vi "RP read signal channel.vi"(7 "Pipeline delay":dbl=28.0, 8 "Error In":errorcluster, 9 "Channel name":string, 11 "File Path Control":path) -> (0 "Error Out":errorcluster, 1 "Phase":dbl, 2 "Frequency":dbl format="%_19p", 3 "Data out":waveform(dbl), 4 "Phase word":u32, 5 "Frequency word":u32)   [LabVIEW 2015]
panel:
  out "t0":dbl format="%#_6p"
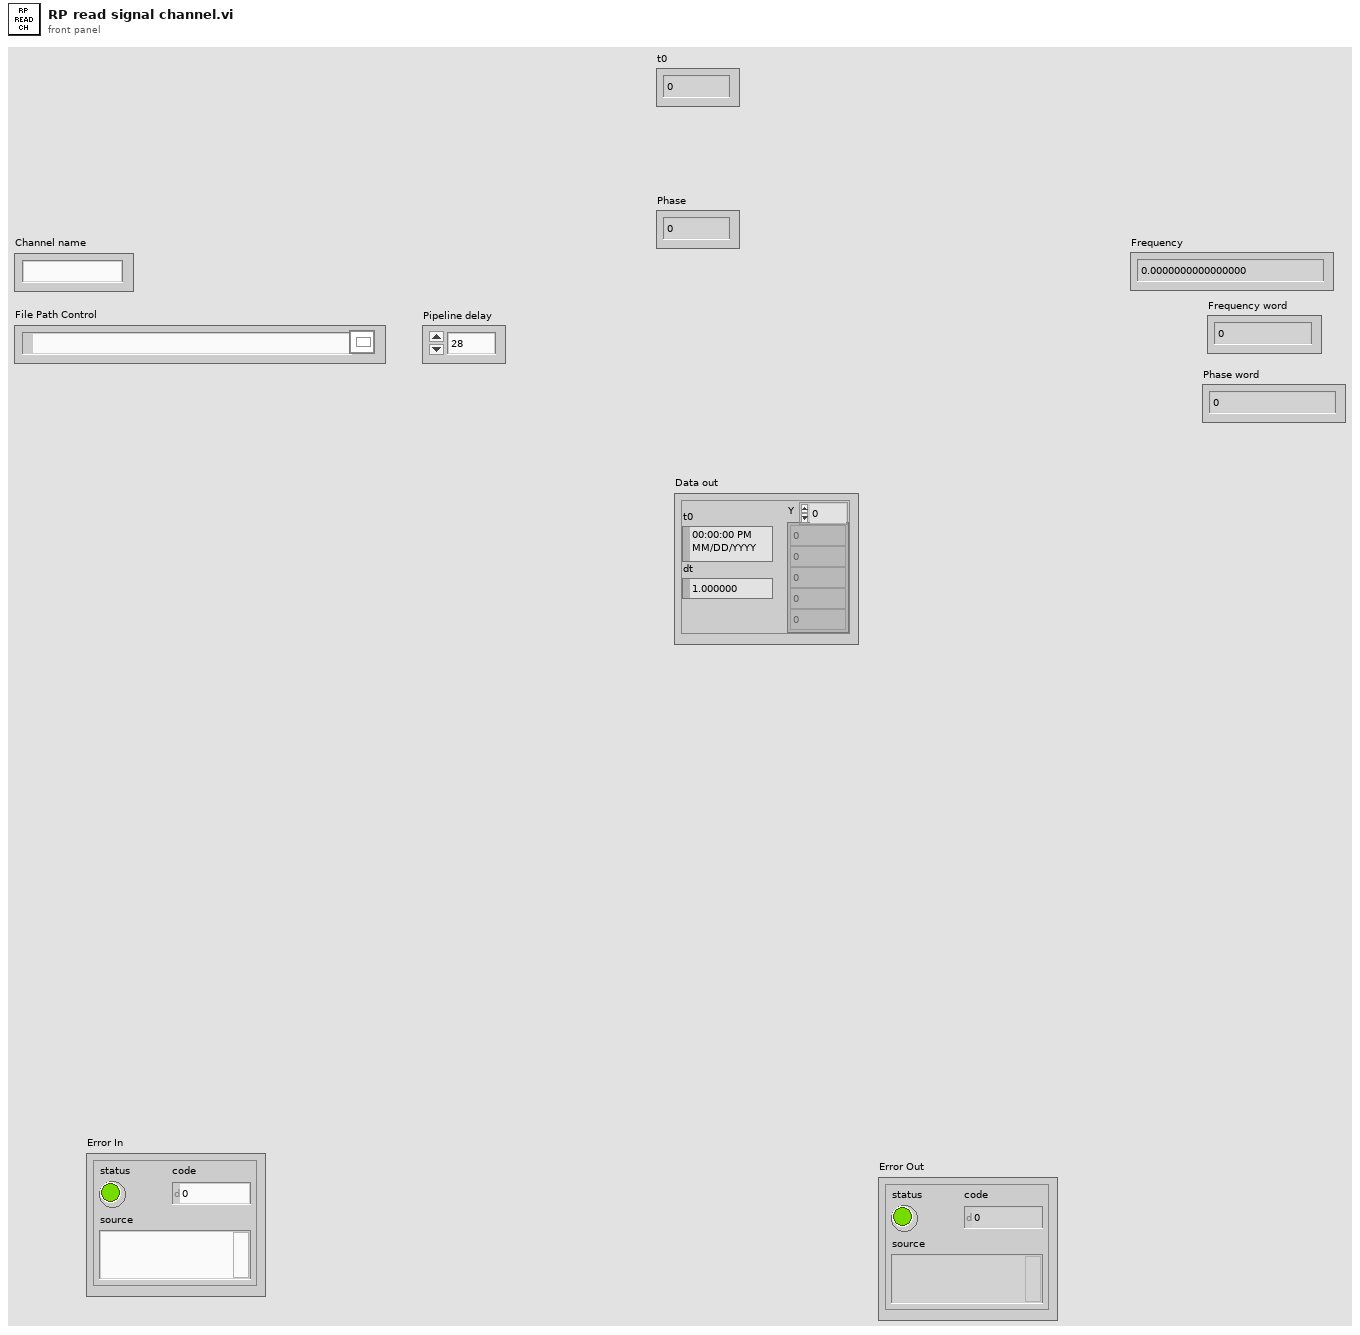
[diagram p1: front panel]
types:
  T1 = enum16{"open", "open or create", "create or replace", "create", "open (read-only)"}
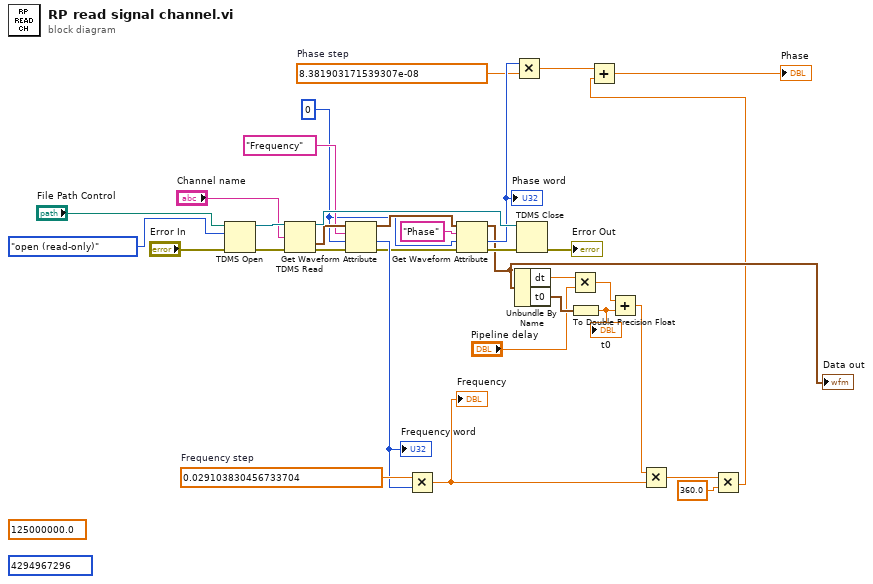
[diagram p0: block diagram]
diagram:
  w7 = u32 0 ("index")
  w23 = 8.381903171539307e-08  # Phase step
  w26 = 0.029103830456733704  # Frequency step
  (unwired) u64 4294967296
  (unwired) 125000000.0
  n1 = TDMS Open(8:"Error In", 10:T1."open (read-only)" ("operation (0:open)"), 11:"File Path Control") -> (0:w30:errorcluster, 3:w29:refnum<k34>)  [unwired: 4 in]
  n2 = TDMS Read(0:w29, 7:"Channel name", 11:w30) -> (4:w28:refnum<k34>, 10:w13:waveform(dbl), 15:w11:errorcluster)  [unwired: 5 in, 3 out]
  n3 = Get Waveform Attribute(4:w11, 5:w7, 6:"Frequency" ("name"), 7:w13) -> (0:w9:errorcluster, 1:w25:u32, 3:w10:waveform(dbl))  [unwired: 1 out]
  "Frequency word" <- w25
  n4 = Multiply(x=w26, y=w25) -> (x*y=w22:dbl)
  "Frequency" <- w22
  n5 = Get Waveform Attribute(4:w9, 5:w7, 6:"Phase" ("name"), 7:w10) -> (0:w27:errorcluster, 1:w24:u32, 3:w4:waveform(dbl))  [unwired: 1 out]
  "Phase word" <- w24
  "Data out" <- w4
  n6 = Multiply(x=w24, y=w23) -> (x*y=w1:dbl)
  n7 = Unbundle By Name(w4) -> ("dt"=w16:dbl, "t0"=w18:timestamp)
  n8 = TDMS Close(8:w27, 11:w28) -> (0:→"Error Out":errorcluster)  [unwired: 1 out]
  n9 = Multiply(x=w16, y="Pipeline delay") -> (x*y=w14:dbl)
  n10 = To Double Precision Float(number=w18) -> (double precision float=w21:dbl)
  "t0" <- w21
  n11 = Add(x=w14, y=w21) -> (x+y=w15:dbl)
  n12 = Multiply(x=w15, y=w22) -> (x*y=w20:dbl)
  n13 = Multiply(x=w20, y=360.0) -> (x*y=w2:dbl)
  n14 = Add(x=w1, y=w2) -> (x+y=→"Phase":dbl)
